vi "Get Program Name.vi"() -> (3 "String":string)   [LabVIEW 2021, in "Logger.lvclass"]
uses:
  Logger.lvclass
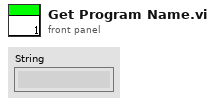
[diagram p1: front panel]
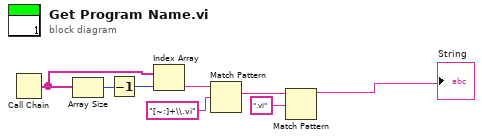
[diagram p0: block diagram]
diagram:
  n1 = Call Chain() -> (call chain=w1:string[])
  n2 = Array Size(array=w1) -> (size(s)=w2:i32)
  n3 = Decrement(x=w2) -> (x-1=w3:i32)
  n4 = Index Array(array=w1, index=w3) -> (element=w4:string)
  n5 = Match Pattern(string=w4, regular expression="[~:]+\\.vi") -> (match substring=w5:string)  [unwired: 1 in, 3 out]
  n6 = Match Pattern(string=w5, regular expression=".vi") -> (before substring=→"String":string)  [unwired: 1 in, 3 out]
